vi "HEWH RLT Compile TCs For Station.vi"(8 "Error In":errorcluster, 9 "Station ID":string="A", 10 "Agilent Cluster Array In":T1[](array[typedef])=[{"Label"="T1-17", "Agilent Channel"="109", "Panel ID"="", "Source"="", "Temperature"=20.0}, {"Label"="T1-18", "Agilent Channel"="110", "Panel ID"="", "Source"="", "Temperature"=21.0}], 11 "RLT Station Channels In":T2={"MW100"={"Station A Channels, MW100"=[], "Station B Channels, MW100"=[], "Station C Channels, MW100"=[], "Station D Channels, MW100"=[]}, "Agilent"={"Station A Channels, Agilent"=[["T1-17", "109"], ["T1-18", "110"]], "Station B Channels, Agilent"=[], "Station C Channels, Agilent"=[], "Station D Channels, Agilent"=[]}}) -> (0 "Error Out":errorcluster, 2 "Agilent Cluster Array Out":T1[](array[typedef])=[{"Label"="T1-17", "Agilent Channel"="109", "Panel ID"="", "Source"="", "Temperature"=20.0}, {"Label"="T1-18", "Agilent Channel"="110", "Panel ID"="", "Source"="", "Temperature"=21.0}], 3 "RLT Station Channels Out":T2={"MW100"={"Station A Channels, MW100"=[], "Station B Channels, MW100"=[], "Station C Channels, MW100"=[], "Station D Channels, MW100"=[]}, "Agilent"={"Station A Channels, Agilent"=[["T1-17", "109"], ["T1-18", "110"]], "Station B Channels, Agilent"=[], "Station C Channels, Agilent"=[], "Station D Channels, Agilent"=[]}}, 5 "Data (Label,Data)":string[][](array[string])=[["T1-17", "20.000000"], ["T1-18", "21.000000"]])   [LabVIEW 2023]
uses:
  Type Definitions/HEWH Agilent Cluster.ctl
  Type Definitions/HEWH RLT MW100 Station Channels.ctl
  <vilib>/Utility/error.llb/whitespace.ctl
  <vilib>/Utility/error.llb/Trim Whitespace One-Sided.vi
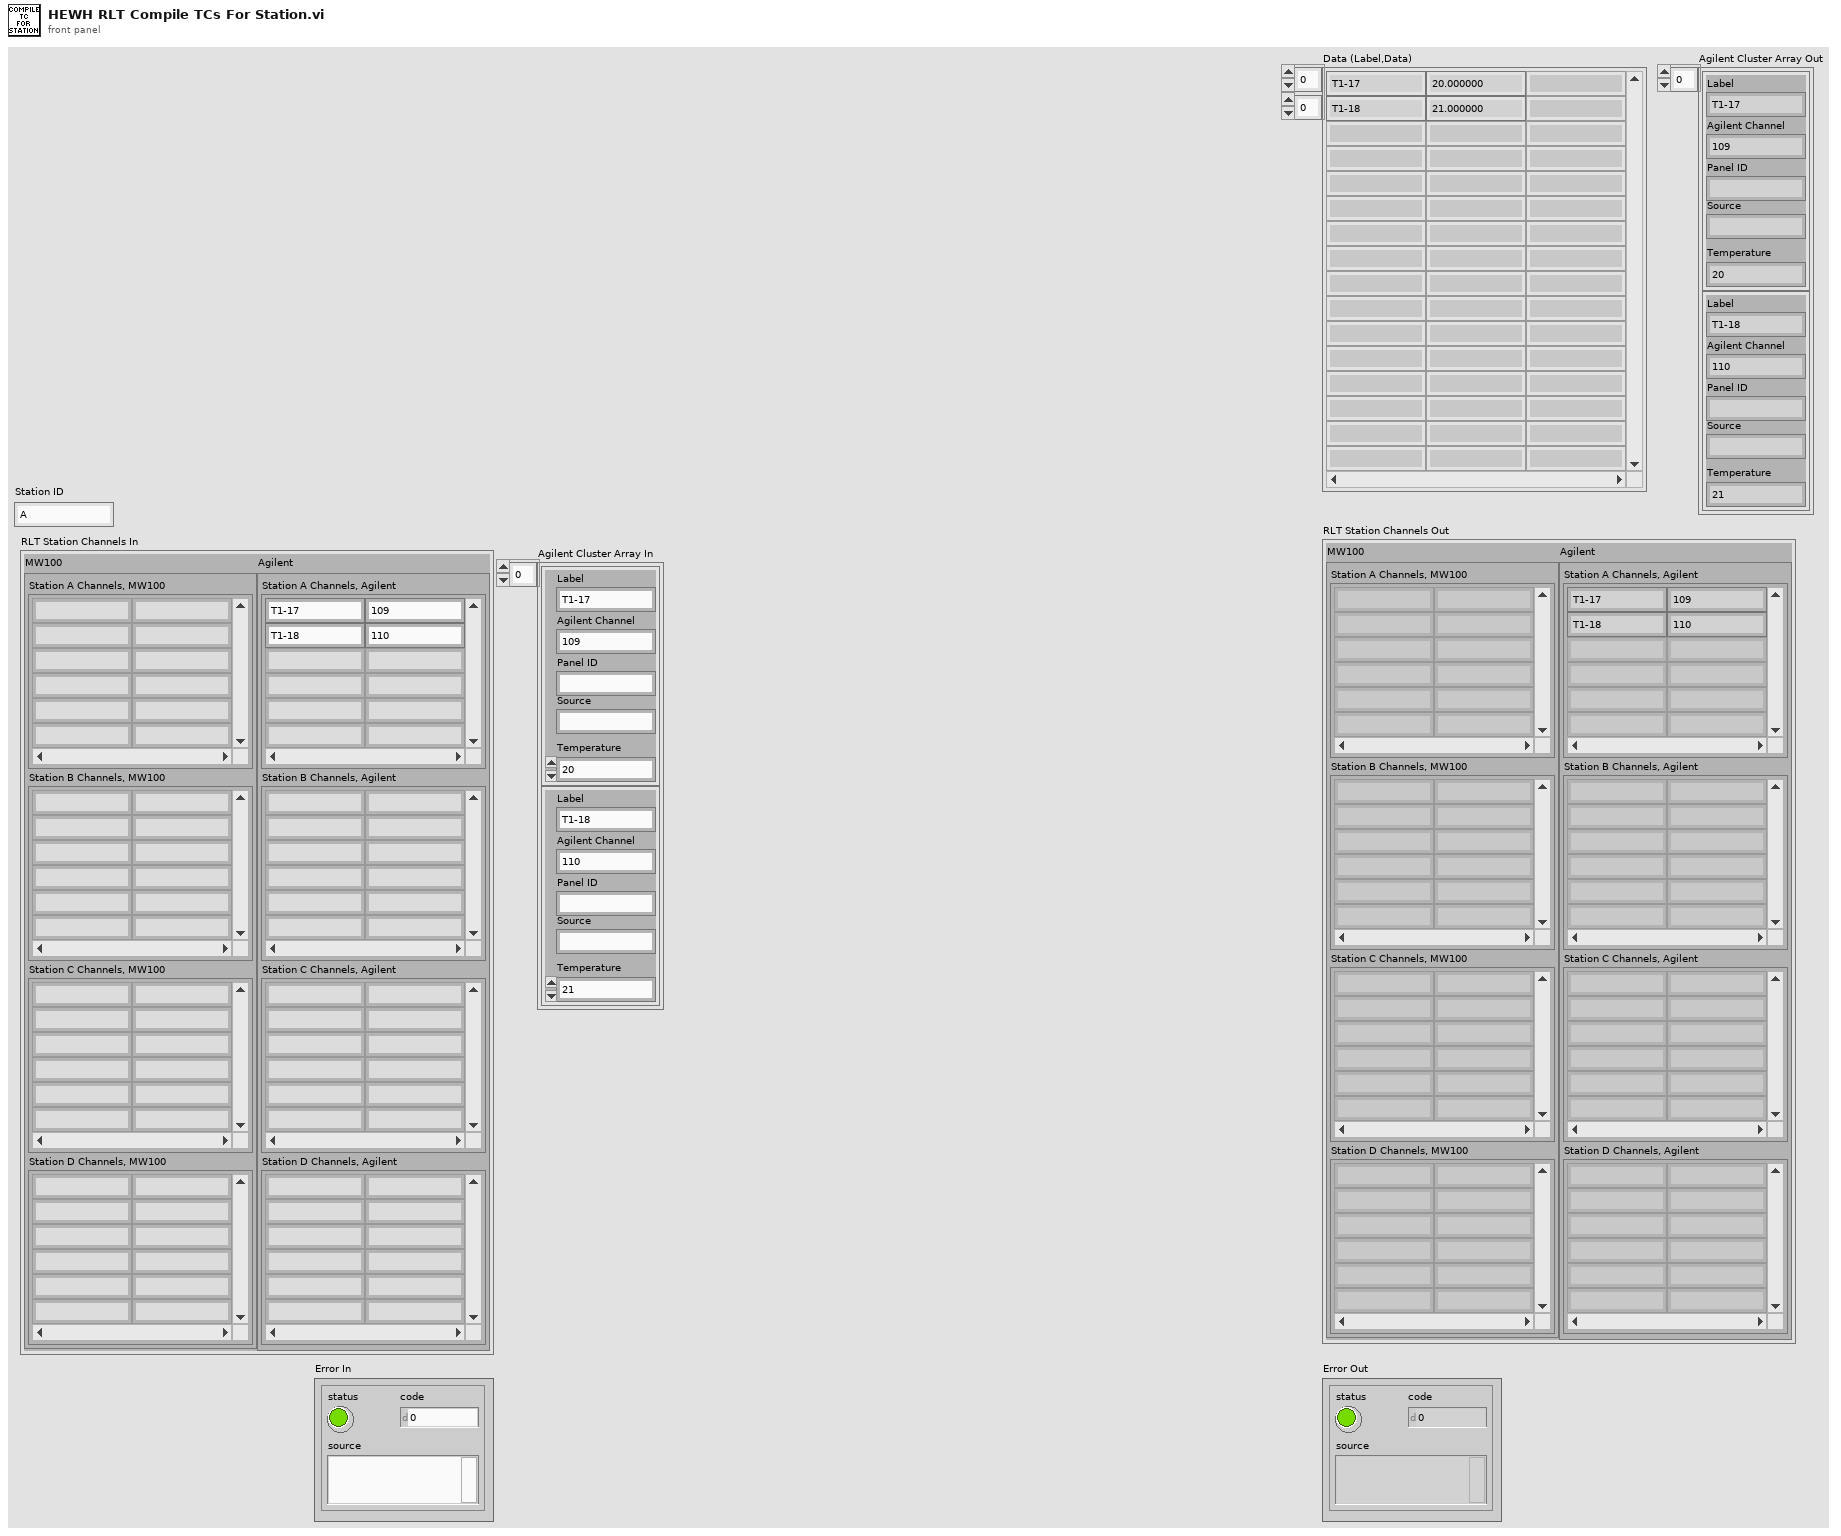
[diagram p1: front panel]
types:
  T1 = typedef "HEWH Agilent Cluster.ctl" = cluster{"Label":string, "Agilent Channel":string, "Panel ID":string, "Source":string, "Temperature":dbl}
  T2 = typedef "HEWH RLT MW100 Station Channels.ctl" = cluster{"MW100":cluster{"Station A Channels, MW100":string[][], "Station B Channels, MW100":string[][], "Station C Channels, MW100":string[][], "Station D Channels, MW100":string[][]}, "Agilent":cluster{"Station A Channels, Agilent":string[][], "Station B Channels, Agilent":string[][], "Station C Channels, Agilent":string[][], "Station D Channels, Agilent":string[][]}}
  T3 = typedef "whitespace.ctl" = u16
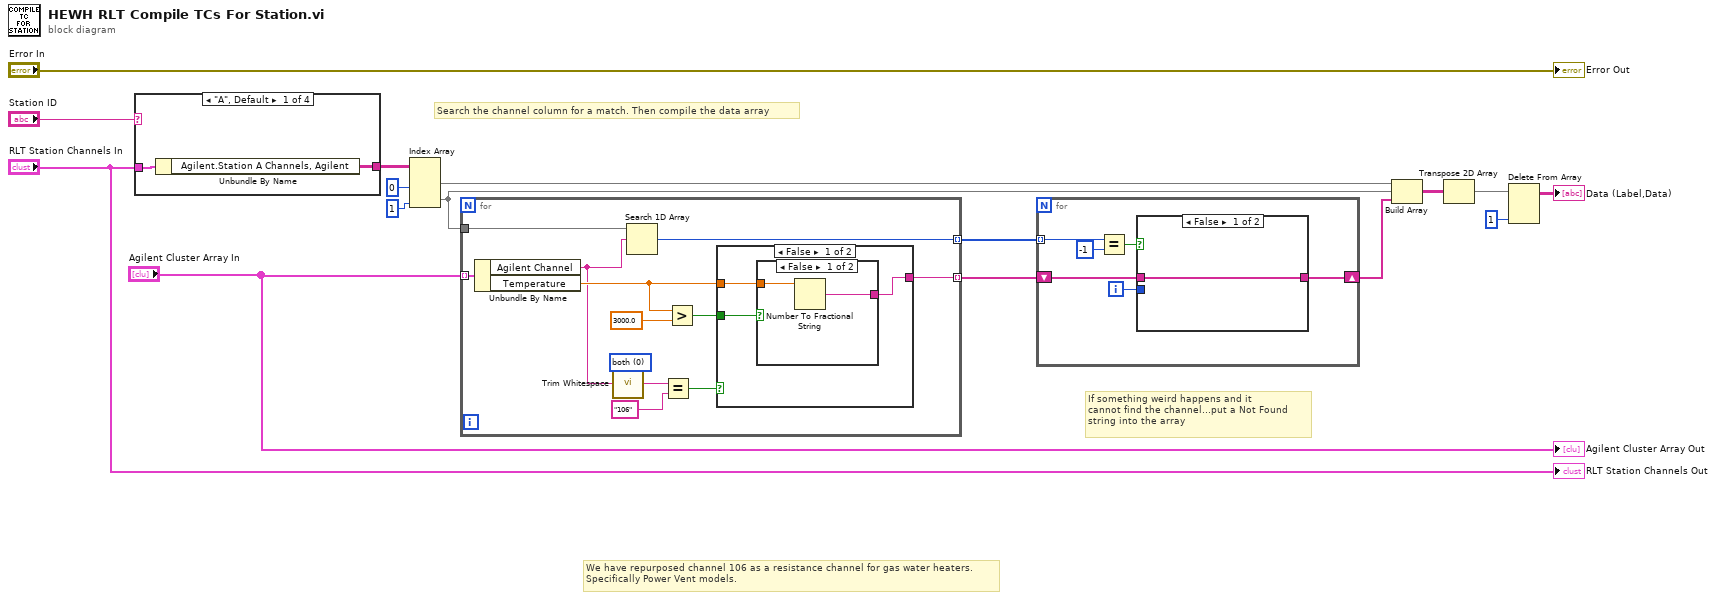
[diagram p0: block diagram]
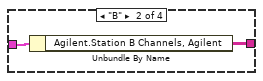
[diagram p2: hidden frame]
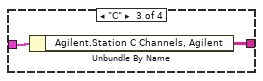
[diagram p3: hidden frame]
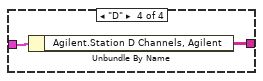
[diagram p4: hidden frame]
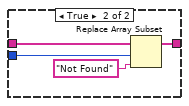
[diagram p5: hidden frame]
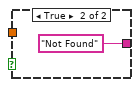
[diagram p6: hidden frame]
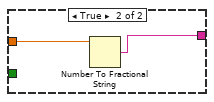
[diagram p7: hidden frame]
diagram:
  # "We have repurposed channel 106 as a resistance channel for gas water heaters.\nSpecifically Power Vent models."
  # "If something weird happens and it \ncannot find the channel...put a Not Found\nstring into the array"
  # "Search the channel column for a match. Then compile the data array"
  n1 = case shown="\"A\", Default" "Station ID" {
    tunnel: "RLT Station Channels In" -> [w18 w20 w22 w24]
    tunnel: [w17 w19 w21 w23] -> w4
    frame "A", Default {
      n2 = Unbundle By Name(w18) -> ("Agilent.Station A Channels, Agilent"=w17:string[][])
    }
    frame "B" {
      n3 = Unbundle By Name(w20) -> ("Agilent.Station B Channels, Agilent"=w19:string[][])
    }
    frame "C" {
      n4 = Unbundle By Name(w22) -> ("Agilent.Station C Channels, Agilent"=w21:string[][])
    }
    frame "D" {
      n5 = Unbundle By Name(w24) -> ("Agilent.Station D Channels, Agilent"=w23:string[][])
    }
  }
  n6 = Index Array(array=w4, index (col) #1=0 ("disabled index (col)"), index (col) #2=1 ("disabled index (col)")) -> (element #1=w8:string[], element #2=w7:string[])  [unwired: 2 in]
  n7 = for {
    tunnel: "Agilent Cluster Array In" -> [w36] mode=indexing
    tunnel: w7 -> [w35]
    tunnel: [w34] -> w13 mode=indexing
    tunnel: [w33] -> w12 mode=indexing
    w28 = T3 0 items=["both", "start of string", "end of string"] ("location (both)")
    n8 = Unbundle By Name(w36) -> ("Agilent Channel"=w29:string, "Temperature"=w32:dbl)
    n9 = call <vilib>:"Trim Whitespace.vi"("string"=w29, "location (both)"=w28) -> ("trimmed string"=w27:string)
    n10 = Search 1D Array(1D array=w35, element=w29) -> (index of element=w34:i32)  [unwired: 1 in]
    n11 = Equal?(x=w27, y="106") -> (x = y?=w25:bool)
    n12 = Greater?(x=w32, y=3000.0) -> (0:w30:bool)
    n13 = case shown="False" w25 {
      tunnel: [w39 w43] -> w33
      tunnel: w32 -> [w38 w44]
      tunnel: w30 -> [w37 _]
      frame False {
        n14 = case shown="False" w37 {
          tunnel: [w41 "Not Found"] -> w39
          tunnel: w38 -> [w40 _]
          frame False {
            n15 = Number To Fractional String(number=w40) -> (F-format string=w41:string)  [unwired: 3 in]
          }
          frame True {
          }
        }
      }
      frame True {
        n16 = Number To Fractional String(number=w44) -> (F-format string=w43:string)  [unwired: 3 in]
      }
    }
  }
  n17 = for {
    tunnel: w13 -> [w50] mode=indexing
    shift-right: [w45] -> w11
    shift-left: w12 -> [w47]
    i -> [w46]
    n18 = Equal?(x=w50, y=-1) -> (x = y?=w48:bool)
    n19 = case shown="False" w48 {
      tunnel: w47 -> [w51 w55]
      tunnel: w46 -> [_ w53]
      tunnel: [w51 w52] -> w45
      frame False {
      }
      frame True {
        n20 = Replace Array Subset(array=w55, new element="Not Found", index=w53) -> (w52:string[])
      }
    }
  }
  n21 = Build Array(w8, w7, w11) -> (w14:string[][])
  n22 = Transpose 2D Array(2D array=w14) -> (transposed array=w3:string[][])
  n23 = Delete From Array(array=w3, index (col)=1 ("index (row)")) -> (array with subset deleted=→"Data (Label,Data)":string[][])  [unwired: 2 in, 1 out]
  "Error Out" <- "Error In"
  "RLT Station Channels Out" <- "RLT Station Channels In"
  "Agilent Cluster Array Out" <- "Agilent Cluster Array In"
